vi "reenvioBloqueoSMS (SubVI).vi"(10 "Datos":T1={"Imei"="356895033079396", "Evento"="359772033694416", "Lat"="359772033694416", "Lon"="359772033694416", "F_H_eve"=timestamp(0 s since 1904-01-01), "F_H_rec"=timestamp(0 s since 1904-01-01)}) -> ()   [LabVIEW 2012]
uses:
  <vilib>/addons/database/Auxilliary.llb/DB Tools Cursor Type.ctl
  <vilib>/addons/database/Connection.llb/DB Tools Open Connec (Path).vi
  <vilib>/addons/database/Connection.llb/Conn Execute.vi
  <vilib>/addons/database/Recordset.llb/Rec Get Recordset Properties (R).vi
  <vilib>/addons/database/Recordset.llb/Rec Fetch String Data (R).vi
  <vilib>/addons/database/Recordset.llb/Rec Destroy - Connection.vi
  <vilib>/addons/database/NI_Database_API.lvlib
panel:
  in  "VISA resource name":refnum<visa-resource-name>="COM17"
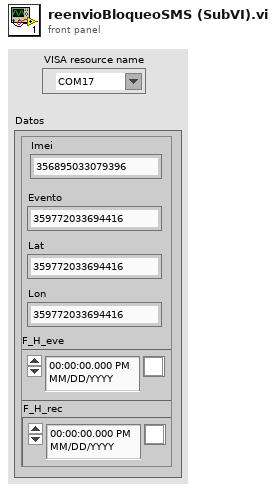
[diagram p1: front panel]
types:
  T1 = cluster{"Imei":string, "Evento":string, "Lat":string, "Lon":string, "F_H_eve":timestamp, "F_H_rec":timestamp}
  T2 = cluster{"VISA resource name":refnum<visa-resource-name>, "Pass":string, "NUMERO":string}
  T3 = typedef "NI_Database_API.lvlib/DB Tools Cursor Type.ctl" = enum16{"forward-only", "keyset", "dynamic", "static"}
  T4 = enum16{"POC", "Imei", "Evento", "Lat", "Lon", "F_H_eve", "F_H_rec", "AVL_N", "AVL_pass", "Propietario", "Razon_Social", "Direccion", "Propietario_N", "Ciudad", "Marca", "Ruta", "N_Ruta", "Auditor", "Auditor_N"}
  T5 = typedef "NI_Database_API.lvlib/Conn ObjectReference.ctl" = refnum<k1>
  T6 = typedef "NI_Database_API.lvlib/Rec ObjectReference.ctl" = refnum<k1>
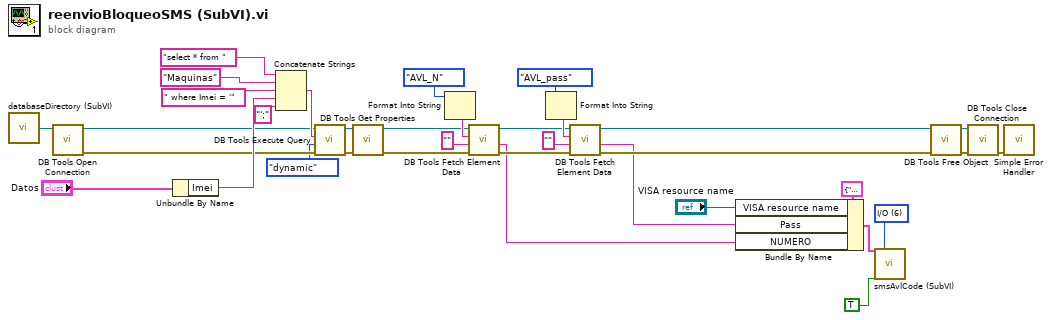
[diagram p0: block diagram]
diagram:
  w9 = u16 6 items=["Password", "APN", "IP/Port", "DNS", "GPRS", "Intervalo", "I/O"] ("Comando")
  n1 = call "databaseDirectory (SubVI).vi"() -> ("Application Directory"=w22:path)  [unwired: 1 in]
  n2 = call-poly <vilib>:"DB Tools Open Connection.vi"("connection information"=w22) -> ("error out"=w18:errorcluster, "connection reference"=w19:T5)  [unwired: 7 in]
  n3 = Unbundle By Name("Datos") -> ("Imei"=w20:string)
  n4 = Concatenate Strings("select * from " ("SQL query"), "Maquinas" ("table"), " where Imei = '" ("Substring"), w20, "';") -> (w30:string)
  n5 = call-poly <vilib>:"DB Tools Execute Query.vi"("error in (no error)"=w18, "cursor type"=DB_Tools_Cursor_Type."dynamic", "SQL query"=w30, "connection reference"=w19) -> ("error out"=w31:errorcluster, "recordset reference"=w32:T6)  [unwired: 4 in]
  n6 = call-poly <vilib>:"DB Tools Get Properties.vi"("error in (no error)"=w31, "recordset reference"=w32) -> ("error out"=w2:errorcluster, "recordset reference out"=w3:T6)  [unwired: 3 in, 1 out]
  n7 = Format Into String(T4."AVL_N") -> (resulting string=w25:string)  [unwired: 3 in, 1 out]
  n8 = call-poly <vilib>:"DB Tools Fetch Element Data.vi"("error in (no error)"=w2, "type"="", "column index"=w25, "recordset reference"=w3) -> ("error out"=w13:errorcluster, "data"=w4:string, "recordset reference out"=w14:T6)  [unwired: 3 in]
  n9 = Format Into String(T4."AVL_pass") -> (resulting string=w15:string)  [unwired: 3 in, 1 out]
  n10 = call-poly <vilib>:"DB Tools Fetch Element Data.vi"("error in (no error)"=w13, "type"="", "column index"=w15, "recordset reference"=w14) -> ("error out"=w11:errorcluster, "data"=w5:string, "recordset reference out"=w12:T6)  [unwired: 3 in]
  n11 = Bundle By Name(cluster=T2 {"VISA resource name"="", "Pass"="", "NUMERO"=""} ("Iniciar"), "VISA resource name"="VISA resource name", "Pass"=w5, "NUMERO"=w4) -> (w8:T2)
  n12 = call "smsAvlCode (SubVI).vi"("Iniciar"=w8, "I/O"=TRUE, "Comando"=w9) -> ()  [unwired: 25 in]
  n13 = call-poly <vilib>:"DB Tools Free Object.vi"("error in (no error)"=w11, "recordset reference"=w12) -> ("error out"=w34:errorcluster, "connection reference"=w33:T5)  [unwired: 8 in]
  n14 = call <vilib>:"DB Tools Close Connection.vi"("error in (no error)"=w34, "connection reference"=w33) -> ("error out"=w35:errorcluster)  [unwired: 5 in]
  n15 = call <vilib>:"Simple Error Handler.vi"("error in (no error)"=w35) -> ()  [unwired: 4 in, 5 out]
